vi "SbigSetTemp.vi"(4 "Temp Regulation":T1 {"CCD Set Point" format="%.2f"; "Auto Freeze" items=["AUTO ON", "AUTO OFF"]; "Regulation" items=["OFF", "ON", "OVERRIDE"]}, 5 "SbigReference":T2, 6 "error in (no error)":errorcluster) -> (0 "error out":errorcluster)   [LabVIEW 2009]
uses:
  Controls/SbigReference.ctl
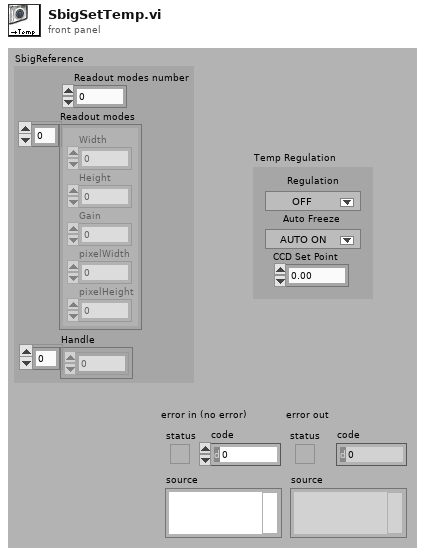
[diagram p1: front panel]
types:
  T1 = cluster{"Regulation":u16, "Auto Freeze":u16, "CCD Set Point":dbl}
  T2 = typedef "SbigReference.ctl" = cluster{"Readout modes number":u16, "Readout modes":cluster{"Width":u16, "Height":u16, "Gain":dbl, "pixelWidth":dbl, "pixelHeight":dbl}[], "Handle":u16[]}
  T3 = enum16{"0-NoCommand", "1-StartExposure", "2-EndExposure", "3-ReadoutLine", "4-DumpLines", "5-SetTemperatureRegulation", "6-QueryTemperatureStatus", "7-ActivateRelay", "8-PulseOut", "9-EstablishLink", "10-GetDriverInfo", "11-GetCCDInfo", "12-QueryCommandStatus", "13-MiscellaneousControl", "14-ReadSubstractLine", "15-UpdateClock", "16-ReadOffset", "17-OpenDriver", "18-CloseDriver", "19-TXSerialBytes", "20-GetSerialStatus", "21-AOTipTilt", "22-AOSetFocus", "23-AODelay", "24-GetTurboStatus", "25-EndReadout", "26-GetUSTimer", "27-OpenDevice", "28-CloseDevice", "29-SetIRQL", "30-GetIRQL", "31-GetLine", "32-GetLinkStatus", "33-GetDriverHandle", "34-SetDriverHandle", "35-StartReadout", "36-GetErrorString", "37-SetDriverControl", "38-GetDriverControl", "39-USBADControl", "40-QueryUSB", "41-GetPentiumCycleCount", "42-RWUSBI2C", "43-CFW"}
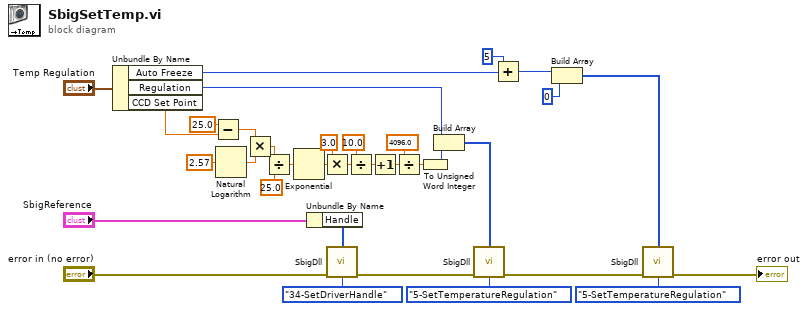
[diagram p0: block diagram]
diagram:
  n1 = Unbundle By Name("Temp Regulation") -> ("Auto Freeze"=w2:u16, "Regulation"=w4:u16, "CCD Set Point"=w3:dbl)
  n2 = Subtract(x=25.0, y=w3) -> (x-y=w22:dbl)
  n3 = Natural Logarithm(1:2.57 ("x")) -> (0:w21:dbl)
  n4 = Multiply(x=w22, y=w21) -> (x*y=w14:dbl)
  n5 = Divide(x=w14, y=25.0) -> (x/y=w18:dbl)
  n6 = Exponential(1:w18) -> (0:w17:dbl)
  n7 = Unbundle By Name("SbigReference") -> ("Handle"=w27:u16[])
  n8 = Multiply(x=3.0, y=w17) -> (x*y=w13:dbl)
  n9 = call "SbigDll.vi"("error in (no error)"="error in (no error)", "Command"=T3."34-SetDriverHandle", "Parameters"=w27) -> ("error out"=w30:errorcluster)  [unwired: 1 in, 3 out]
  n10 = Divide(x=10.0, y=w13) -> (x/y=w12:dbl)
  n11 = Increment(x=w12) -> (x+1=w11:dbl)
  n12 = Divide(x=4096.0, y=w11) -> (x/y=w9:dbl)
  n13 = To Unsigned Word Integer(number=w9) -> (unsigned 16bit integer=w8:u16)
  n14 = Build Array(w4, w8) -> (w7:u16[])
  n15 = call "SbigDll.vi"("error in (no error)"=w30, "Command"=T3."5-SetTemperatureRegulation", "Parameters"=w7) -> ("error out"=w29:errorcluster)  [unwired: 1 in, 3 out]
  n16 = Add(x=u16 5, y=w2) -> (x+y=w24:u16)
  n17 = Build Array(w24, u16 0 ("Elément d'entrée")) -> (w6:u16[])
  n18 = call "SbigDll.vi"("error in (no error)"=w29, "Command"=T3."5-SetTemperatureRegulation", "Parameters"=w6) -> ("error out"=→"error out":errorcluster)  [unwired: 1 in, 3 out]
